vi "set backlight.vi"(9 "Disable markers":bool, 10 "Panel Backlight":u8(slide) scale=0.0..10.0, 11 "Array":T1[](array[typedef]) {"Data" format="%.0x"}) -> (3 "Array 2":T1[](array[typedef]) {"Data" format="%.0x"})   [LabVIEW 2021, in "uCanDriver.lvlib" / "uCAN.lvclass"]
uses:
  uCAN.lvclass
  typedefs/frame.ctl
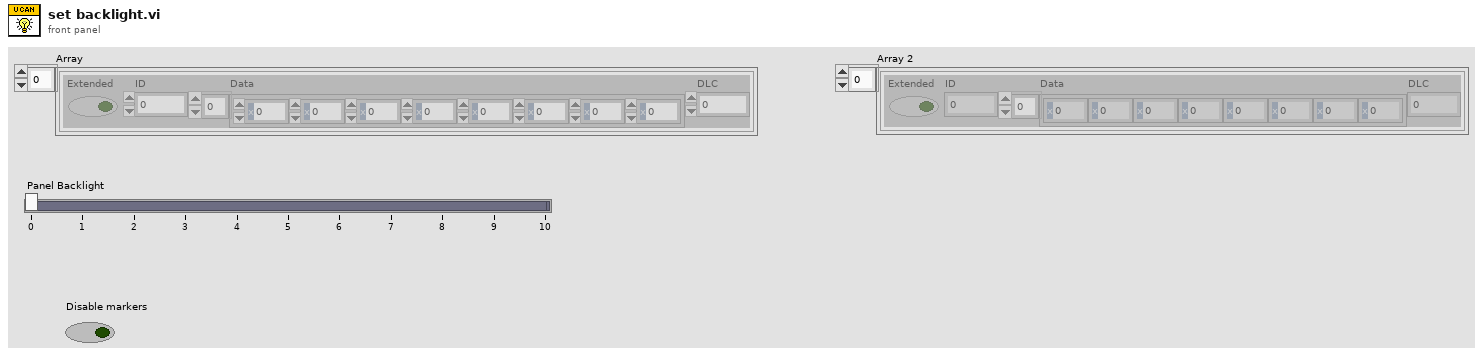
[diagram p1: front panel]
types:
  T1 = typedef "uCanDriver.lvlib/uCAN.lvclass/frame.ctl" = cluster{"Extended":bool, "ID":u32, "Data":u8[], "DLC":u8}
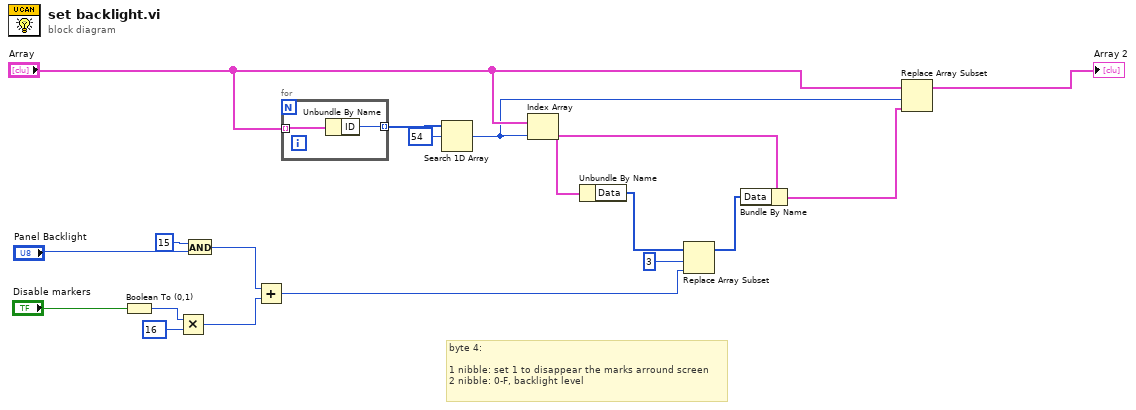
[diagram p0: block diagram]
diagram:
  # "byte 4:\n\n1 nibble: set 1 to disappear the marks arround screen\n2 nibble: 0-F, backlight level"
  n1 = Boolean To (0,1)(Boolean="Disable markers") -> (0, 1=w8:i16)
  n2 = Multiply(x=w8, y=i16 16) -> (x*y=w6:i16)
  n3 = And(x=u8 15, y="Panel Backlight") -> (x .and. y?=w3:u8)
  n4 = Add(x=w3, y=w6) -> (x+y=w2:i16)
  n5 = for {
    tunnel: "Array" -> [w20] mode=indexing
    tunnel: [w19] -> w16 mode=indexing
    n6 = Unbundle By Name(w20) -> ("ID"=w19:u32)
  }
  n7 = Search 1D Array(1D array=w16, element=u32 54) -> (index of element=w14:i32)  [unwired: 1 in]
  n8 = Index Array(array="Array", index=w14) -> (element=w18:T1)
  n9 = Unbundle By Name(w18) -> ("Data"=w11:u8[])
  n10 = Replace Array Subset(array=w11, new element=w2, index=3) -> (w1:u8[])
  n11 = Bundle By Name(cluster=w18, "Data"=w1) -> (w12:T1)
  n12 = Replace Array Subset(array="Array", new element=w12, index=w14) -> (→"Array 2":T1[])
